vi "Update State Data.vi"(8 "error in (no error)":errorcluster, 9 "Data":variant, 10 "Argument":string, 11 "Step in":refnum<class "Step.lvclass">) -> (0 "error out":errorcluster, 3 "Step out":refnum<class "Step.lvclass">)   [LabVIEW 2020, in "MacroAssert.lvlib" / "Step.lvclass"]
uses:
  Step.lvclass
  Step.lvclass/Step.ctl
  MacroAssert.lvlib
  CTLs/Step Type V3.ctl
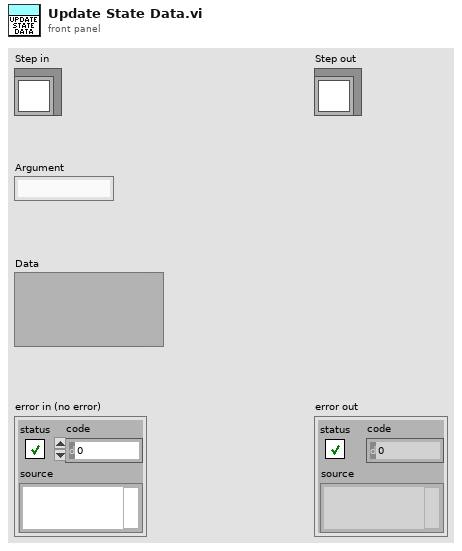
[diagram p1: front panel]
types:
  T1 = typedef "MacroAssert.lvlib/Step Type V3.ctl" = enum16{"Mouse Action", "Keyboard Action", "Window Action", "Timing Action", "Boolean Assertion", "Numeric Assertion", "String Assertion", "Image Assertion"}
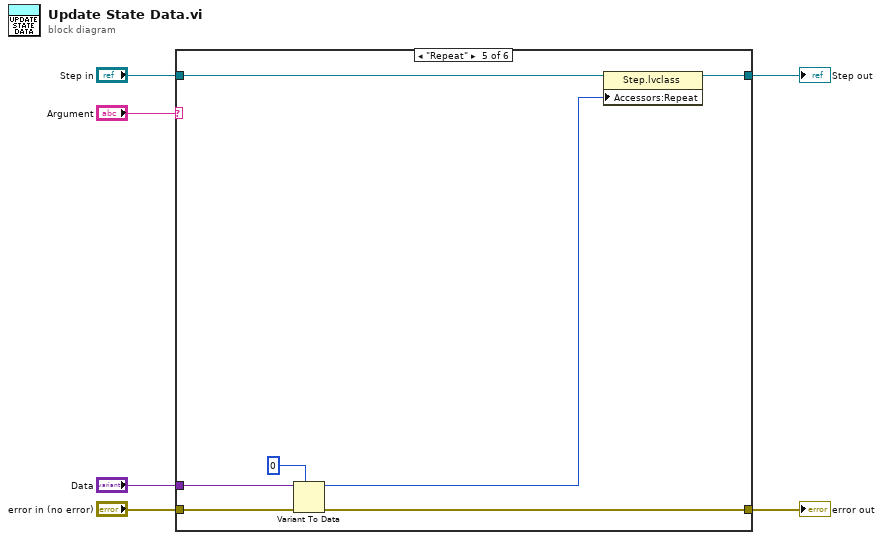
[diagram p0: block diagram]
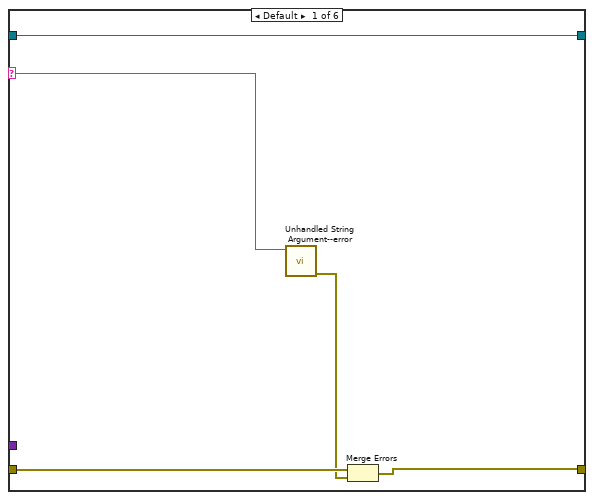
[diagram p2: hidden frame]
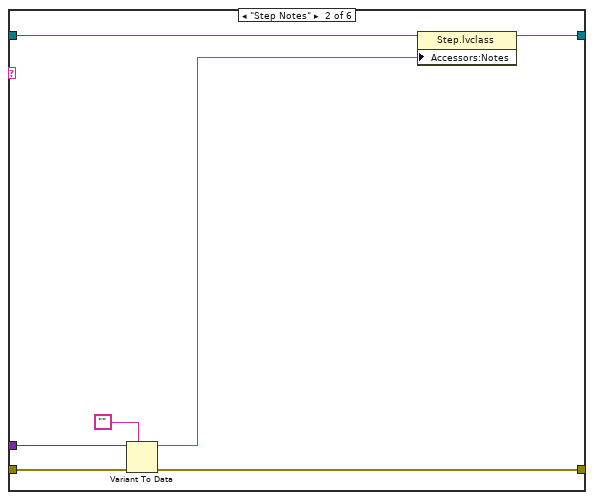
[diagram p3: hidden frame]
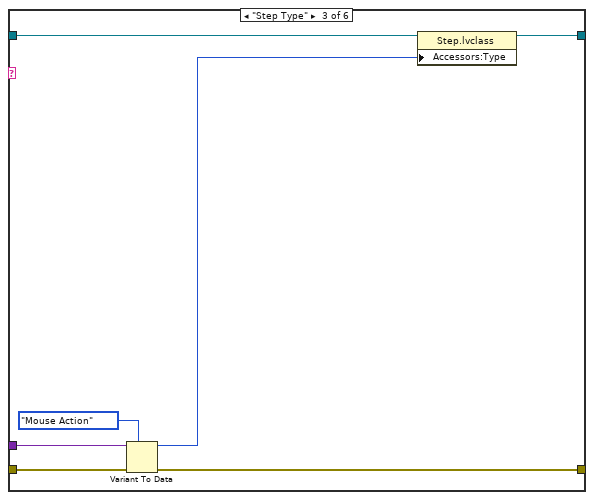
[diagram p4: hidden frame]
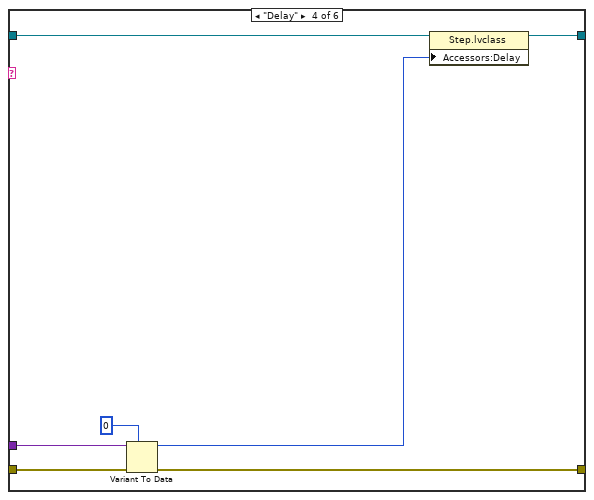
[diagram p5: hidden frame]
diagram:
  n1 = case shown="\"Repeat\"" "Argument" {
    selector: "Argument" -> [w7 _ _ _ _ _]
    tunnel: "Step in" -> [w11 w18 w25 w32 w39 w40]
    tunnel: "error in (no error)" -> [w10 w16 w23 w31 w38 w41]
    tunnel: [w11 w17 w24 w27 w34 w40] -> w3
    tunnel: [w8 w15 w22 w30 w37 w41] -> w6
    tunnel: "Data" -> [_ w14 w21 w29 w36 _]
    frame Default {
      n2 = call "Unhandled String Argument--error.vi"("Argument"=w7) -> ("error out"=w9:errorcluster)  [unwired: 10 in]
      n3 = Merge Errors(w10, w9) -> (w8:errorcluster)
    }
    frame "Step Notes" {
      n4 = Variant To Data(error in=w16, type="", Variant=w14) -> (data=w13:string, error out=w15:errorcluster)
      n5 = property class="Step.lvclass"(reference=w18, "Accessors:Notes"=w13) -> (reference out=w17:refnum<class "Step.lvclass">)  [unwired: 1 in, 1 out]
    }
    frame "Step Type" {
      n6 = Variant To Data(error in=w23, type=Step_Type_V3."Mouse Action" ("Step Type"), Variant=w21) -> (data=w19:T1, error out=w22:errorcluster)
      n7 = property class="Step.lvclass"(reference=w25, "Accessors:Type"=w19) -> (reference out=w24:refnum<class "Step.lvclass">)  [unwired: 1 in, 1 out]
    }
    frame "Delay" {
      n8 = Variant To Data(error in=w31, type=0, Variant=w29) -> (data=w26:i32, error out=w30:errorcluster)
      n9 = property class="Step.lvclass"(reference=w32, "Accessors:Delay"=w26) -> (reference out=w27:refnum<class "Step.lvclass">)  [unwired: 1 in, 1 out]
    }
    frame "Repeat" {
      n10 = Variant To Data(error in=w38, type=0, Variant=w36) -> (data=w33:i32, error out=w37:errorcluster)
      n11 = property class="Step.lvclass"(reference=w39, "Accessors:Repeat"=w33) -> (reference out=w34:refnum<class "Step.lvclass">)  [unwired: 1 in, 1 out]
    }
    frame "Cancel", "OK" {
    }
  }
  "error out" <- w6
  "Step out" <- w3
